vi "_initFileContentsTree.vi"(4 "error in (no error)":errorcluster, 5 "File refnum in":refnum<k20>, 7 "reference":refnum<vi>) -> (0 "error out":errorcluster)   [LabVIEW 2020]
doc: "Initializes a Tree Control with the contents of the input file"
uses:
  <vilib>/Platform/storage/Storage.llb/Get Property (String).vi
  <vilib>/Platform/storage/Storage.llb/Get Property (Storage Refnums).vi
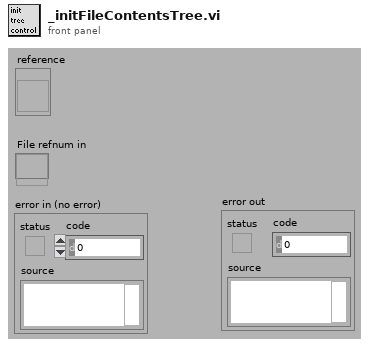
[diagram p1: front panel]
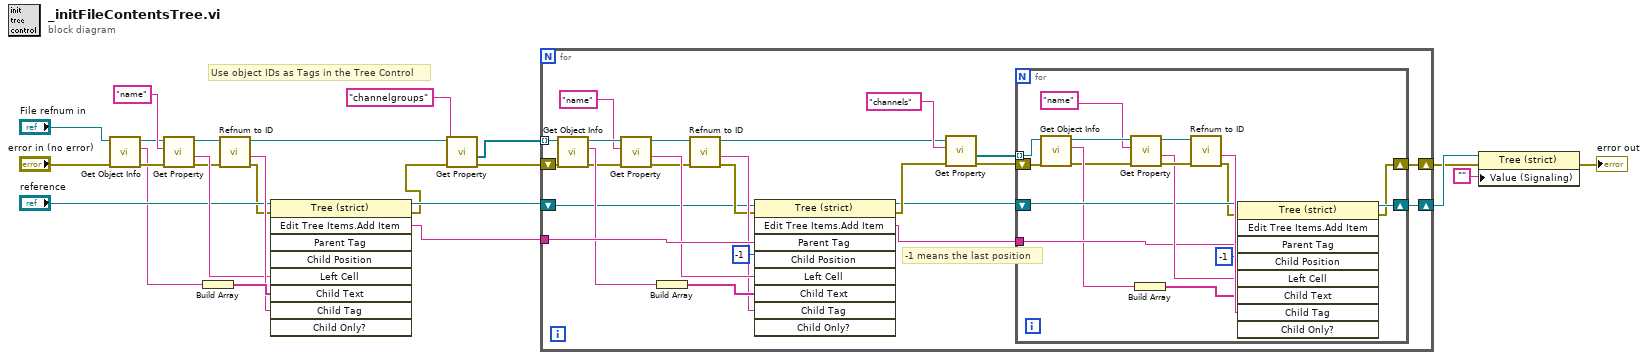
[diagram p0: block diagram]
diagram:
  # "Use object IDs as Tags in the Tree Control"
  n1 = call <vilib>:"Get Object Info.vi"("error in (no error)"="error in (no error)", "storage refnum"="File refnum in") -> ("error out"=w7:errorcluster, "object type"=w6:string, "storage refnum out"=w8:refnum<k20>)  [unwired: 7 out]
  n2 = call-poly <vilib>:"Get Property.vi"("error in (no error)"=w7, "Property name"="name" ("Name"), "storage refnum"=w8) -> ("error out"=w20:errorcluster, "Value"=w21:string, "storage refnum out"=w17:refnum<k20>)  [unwired: 6 out]
  n3 = Build Array(w6) -> (w23:string[])
  n4 = call <vilib>:"Refnum to ID.vi"("error in (no error)"=w20, "storage refnum"=w17) -> ("error out"=w16:errorcluster, "object ID"=w22:string, "storage refnum out"=w1:refnum<k20>)  [unwired: 3 out]
  n5 = invoke on="Invoke Node" class="Tree (strict)" method="Edit Tree Items.Add Item"(reference="reference", error in=w16, "Left Cell"=w21, "Child Text"=w23, "Child Tag"=w22) -> (reference out=w15:refnum<vi>, error out=w2:errorcluster, "Edit Tree Items:Add Item"=w24:string)  [unwired: 4 in, 6 out]
  n6 = call-poly <vilib>:"Get Property.vi"("error in (no error)"=w2, "Property name"="channelgroups", "storage refnum"=w1) -> ("error out"=w3:errorcluster, "Value"=w4:refnum<k20>[])  [unwired: 7 out]
  n7 = for {
    tunnel: w4 -> [w39] mode=indexing
    tunnel: w24 -> [w48]
    shift-right: [w29] -> w14
    shift-left: w15 -> [w28]
    shift-right: [w26] -> w11
    shift-left: w3 -> [w38]
    # "-1 means the last position"
    n8 = call <vilib>:"Get Object Info.vi"("error in (no error)"=w38, "storage refnum"=w39) -> ("error out"=w36:errorcluster, "object type"=w37:string, "storage refnum out"=w35:refnum<k20>)  [unwired: 7 out]
    n9 = call-poly <vilib>:"Get Property.vi"("error in (no error)"=w36, "Property name"="name" ("Name"), "storage refnum"=w35) -> ("error out"=w45:errorcluster, "Value"=w47:string, "storage refnum out"=w34:refnum<k20>)  [unwired: 6 out]
    n10 = Build Array(w37) -> (w46:string[])
    n11 = call <vilib>:"Refnum to ID.vi"("error in (no error)"=w45, "storage refnum"=w34) -> ("error out"=w32:errorcluster, "object ID"=w44:string, "storage refnum out"=w33:refnum<k20>)  [unwired: 3 out]
    n12 = invoke on="Invoke Node" class="Tree (strict)" method="Edit Tree Items.Add Item"(reference=w28, error in=w32, "Parent Tag"=w48, "Child Position"=-1, "Left Cell"=w47, "Child Text"=w46, "Child Tag"=w44) -> (reference out=w30:refnum<vi>, error out=w31:errorcluster, "Edit Tree Items:Add Item"=w43:string)  [unwired: 2 in, 6 out]
    n13 = call-poly <vilib>:"Get Property.vi"("error in (no error)"=w31, "Property name"="channels" ("Channels"), "storage refnum"=w33) -> ("error out"=w41:errorcluster, "Value"=w40:refnum<k20>[])  [unwired: 7 out]
    n14 = for {
      tunnel: w43 -> [w60]
      tunnel: w40 -> [w57] mode=indexing
      shift-right: [w52] -> w29
      shift-left: w30 -> [w59]
      shift-right: [w50] -> w26
      shift-left: w41 -> [w56]
      n15 = call <vilib>:"Get Object Info.vi"("error in (no error)"=w56, "storage refnum"=w57) -> ("error out"=w53:errorcluster, "object type"=w55:string, "storage refnum out"=w54:refnum<k20>)  [unwired: 7 out]
      n16 = call-poly <vilib>:"Get Property.vi"("error in (no error)"=w53, "Property name"="name" ("Name"), "storage refnum"=w54) -> ("error out"=w63:errorcluster, "Value"=w61:string, "storage refnum out"=w64:refnum<k20>)  [unwired: 6 out]
      n17 = Build Array(w55) -> (w62:string[])
      n18 = call <vilib>:"Refnum to ID.vi"("error in (no error)"=w63, "storage refnum"=w64) -> ("error out"=w58:errorcluster, "object ID"=w65:string)  [unwired: 4 out]
      n19 = invoke on="Invoke Node" class="Tree (strict)" method="Edit Tree Items.Add Item"(reference=w59, error in=w58, "Parent Tag"=w60, "Child Position"=-1, "Left Cell"=w61, "Child Text"=w62, "Child Tag"=w65) -> (reference out=w52:refnum<vi>, error out=w50:errorcluster)  [unwired: 2 in, 7 out]
    }
  }
  n20 = property class="Tree (strict)"(reference=w14, error in=w11, "Value (Signaling)"="") -> (error out=→"error out":errorcluster)  [unwired: 1 out]
